vi "FindTagMatchesTreeCluster.vi"(9 "TreeCluster":T1(array[cluster]), 11 "NameToFind":string) -> (2 "TreeCluster":T1(array[cluster]), 3 "ResultString":string)   [LabVIEW 2013, in "FindName Task_Manager.lvlib"]
doc: "Find all tags that match name"
uses:
  FindName Task_Manager.lvlib
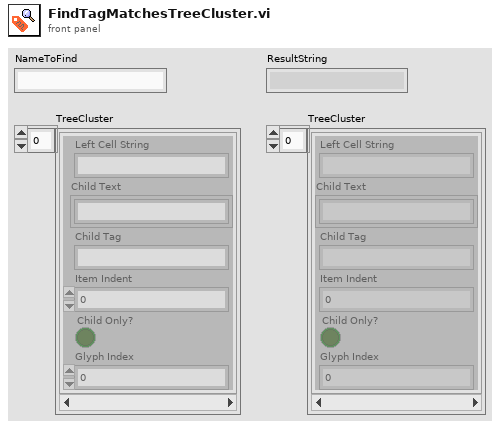
[diagram p1: front panel]
types:
  T1 = cluster{"Left Cell String":string, "Child Text":string[], "Child Tag":string, "Item Indent":i32, "Child Only?":bool, "Glyph Index":i32}[]
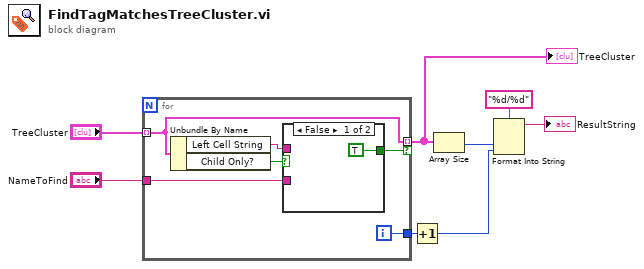
[diagram p0: block diagram]
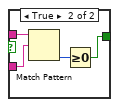
[diagram p2: hidden frame]
diagram:
  n1 = for {
    tunnel: "NameToFind" -> [w14]
    tunnel: "TreeCluster" -> [w13] mode=indexing
    tunnel: [w10] -> w3
    tunnel: [w13] -> w2 mode=indexing if=w12
    i -> [w10]
    n2 = Unbundle By Name(w13) -> ("Left Cell String"=w11:string, "Child Only?"=w9:bool)
    n3 = case shown="False" w9 {
      tunnel: w14 -> [_ w19]
      tunnel: [TRUE w17] -> w12
      tunnel: w11 -> [_ w16]
      frame False {
      }
      frame True {
        n4 = Match Pattern(string=w16, regular expression=w19) -> (offset past match=w18:i32)  [unwired: 1 in, 3 out]
        n5 = Greater Or Equal To 0?(x=w18) -> (x >= 0?=w17:bool)
      }
    }
  }
  "TreeCluster" <- w2
  n6 = Increment(x=w3) -> (x+1=w1:i32)
  n7 = Array Size(array=w2) -> (size(s)=w8:i32)
  n8 = Format Into String(format string="%d/%d", w8, w1) -> (resulting string=→"ResultString":string)  [unwired: 2 in, 1 out]
